vi "队列全变量.vi"() -> ()   [LabVIEW 2011]
panel:
  out "元素":i32
  in  "数值":i32
  in  "方式":enum16{"读队列", "写队列", "释放队列"}(ring)
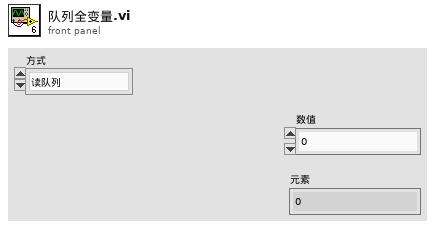
[diagram p1: front panel]
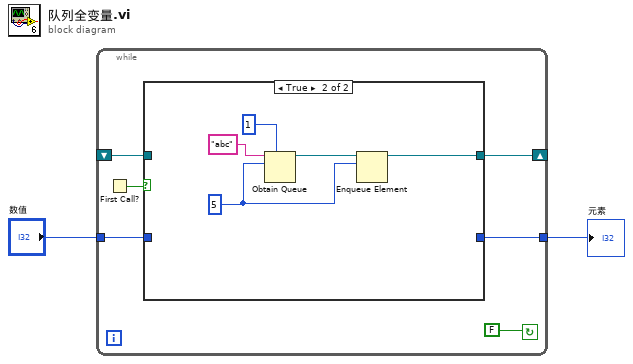
[diagram p0: block diagram]
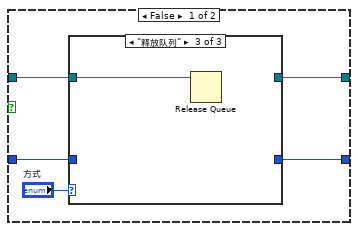
[diagram p2: hidden frame]
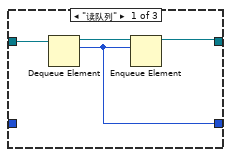
[diagram p3: hidden frame]
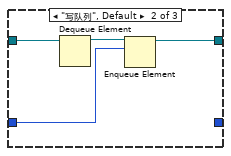
[diagram p4: hidden frame]
diagram:
  n1 = while {
    shift-right: [w6] -> _
    shift-left: _ -> [w5]
    tunnel: "数值" -> [w4]
    tunnel: [w3] -> w1
    stop <- FALSE ("stop") continue-if-true
    n2 = First Call?() -> (First Call?: T/F=w8:bool)
    n3 = case shown="True" w8 {
      tunnel: [w11 w23] -> w6
      tunnel: w5 -> [w12 _]
      tunnel: w4 -> [w10 _]
      tunnel: [w9 _] -> w3
      frame False {
        n4 = case shown="\"释放队列\"" "方式" {
          tunnel: w12 -> [w17 w20 w22]
          tunnel: [w15 w21 _] -> w11
          tunnel: w10 -> [_ w18 _]
          tunnel: [w14 _ _] -> w9
          frame "读队列" {
            n5 = Dequeue Element(queue=w17) -> (queue out=w16:refnum<queue>, element=w14:i32)  [unwired: 2 in, 2 out]
            n6 = Enqueue Element(queue=w16, element=w14) -> (queue out=w15:refnum<queue>)  [unwired: 2 in, 2 out]
          }
          frame "写队列", Default {
            n7 = Dequeue Element(queue=w20) -> (queue out=w19:refnum<queue>)  [unwired: 2 in, 3 out]
            n8 = Enqueue Element(queue=w19, element=w18) -> (queue out=w21:refnum<queue>)  [unwired: 2 in, 2 out]
          }
          frame "释放队列" {
            n9 = Release Queue(queue=w22) -> ()  [unwired: 2 in, 3 out]
          }
        }
      }
      frame True {
        w24 = 5 ("max queue size (-1, unlimited)")
        n10 = Obtain Queue(max queue size (-1, unlimited)=1, name (unnamed)="abc", element data type=w24) -> (queue out=w27:refnum<queue>)  [unwired: 2 in, 2 out]
        n11 = Enqueue Element(queue=w27, element=w24) -> (queue out=w23:refnum<queue>)  [unwired: 2 in, 2 out]
      }
    }
  }
  "元素" <- w1
